vi "vector space kNN.vi"() -> ()   [LabVIEW 2014]
panel:
  out "Numeric":i32
  out "size(s) 2":i32
  out "Results":string[][](array[string])
  out "accuracy":string[][](array[string])
  out "size(s)":i32
  out "Array":string[][](array[string])
  out "appended array":string[](array[string])
  in  "kNN k":i32=5
  out "subarray":dbl[](array[numeric])
  in  "all rows":string[][](array[string])=array2038x3[6114 elements]
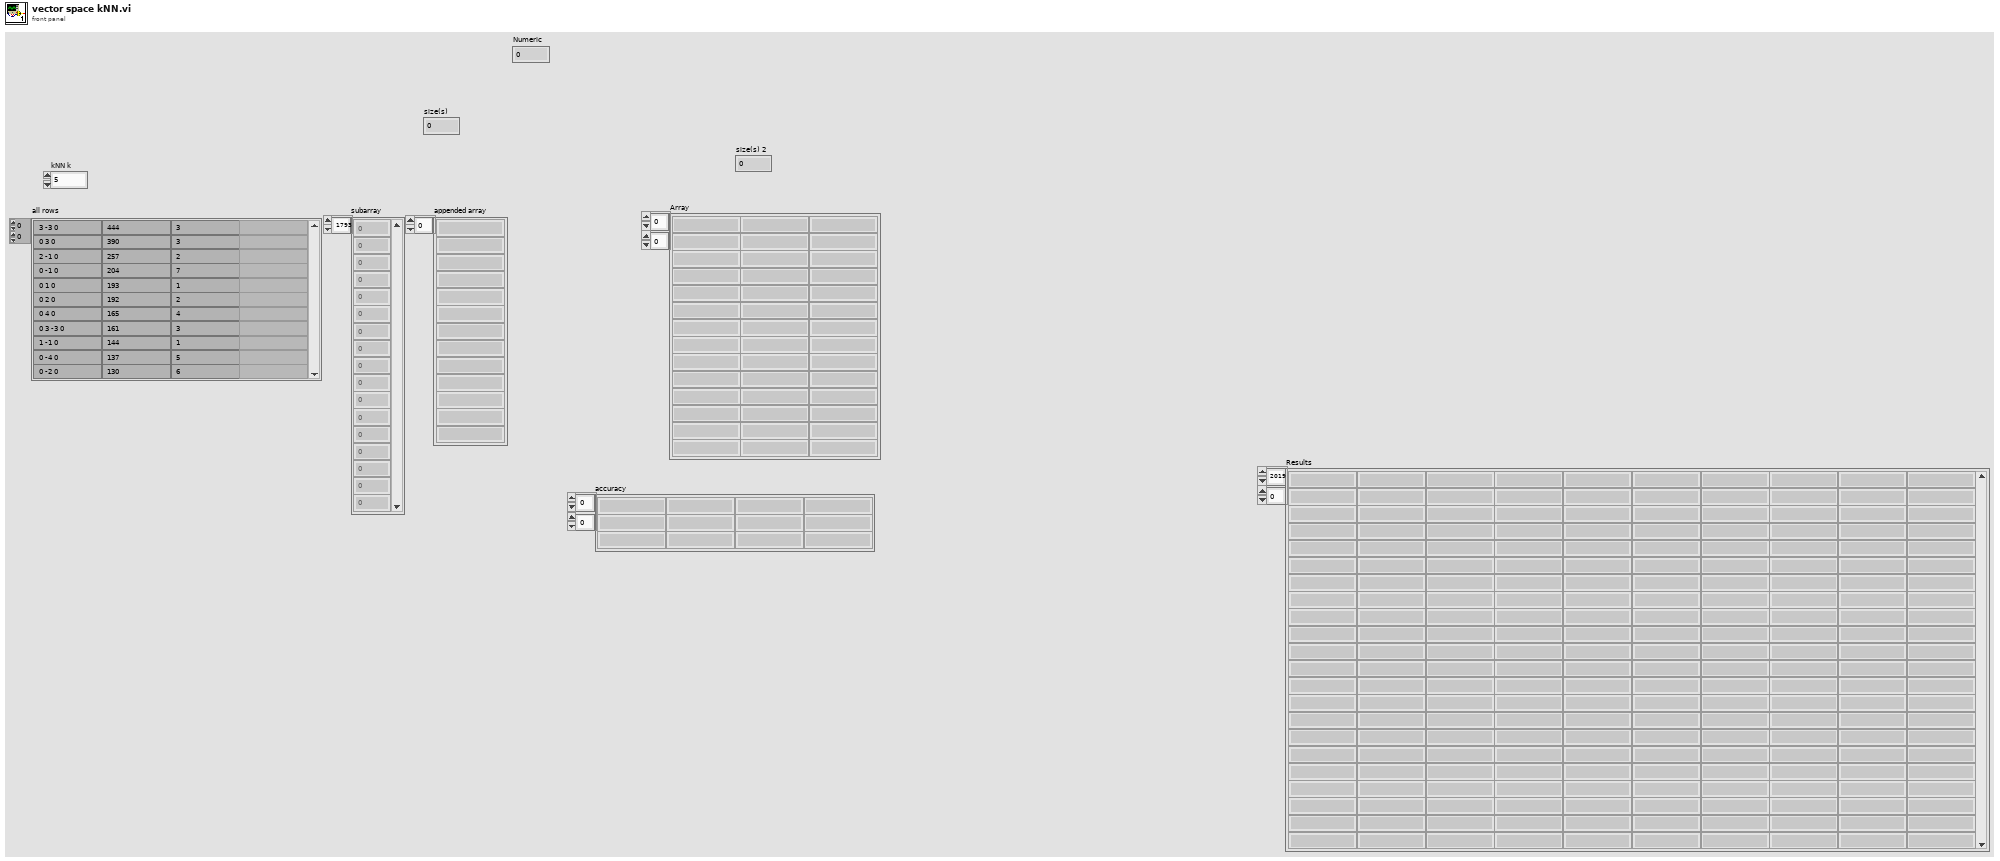
[diagram p1: front panel]
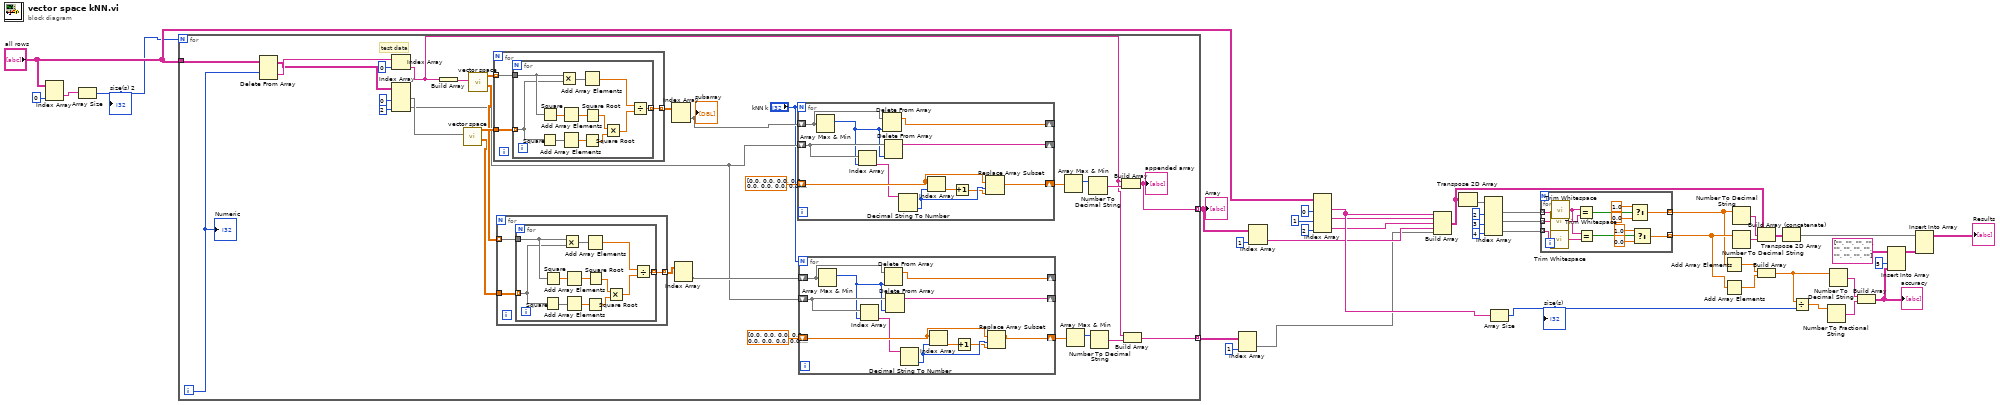
[diagram p0: block diagram]
diagram:
  n1 = Index Array(array="all rows", index (col)=0 ("disabled index (col)")) -> (element=w2:string[])  [unwired: 1 in]
  n2 = Array Size(array=w2) -> (size(s)=w1:i32)
  "size(s) 2" <- w1
  n3 = for {
    N: w1 -> [_]
    tunnel: "all rows" -> [w72]
    tunnel: [w55] -> w9 mode=indexing
    tunnel: [w44] -> w6 mode=indexing
    i -> [w71]
    # "test data"
    n4 = Delete From Array(array=w72, index (row)=w71) -> (deleted portion=w70:string[], array with subset deleted=w67:string[][])  [unwired: 2 in]
    n5 = Index Array(array=w70, index=0 ("disabled index (col)")) -> (element=w45:string)
    n6 = Index Array(array=w67, index (col) #1=0 ("disabled index (col)"), index (col) #2=2 ("index (col)")) -> (element #1=w61:string[], element #2=w46:string[])  [unwired: 2 in]
    n7 = Build Array(w45) -> (w64:string[])
    n8 = call "vector space.vi"("Full transition sequence from service to end"=w61) -> ("vector (directional transitions)"=w52:dbl[][], "vector positions only"=w63:dbl[][])  [unwired: 8 in, 1 out]
    n9 = call "vector space.vi"("Full transition sequence from service to end"=w64) -> ("vector (directional transitions)"=w53:dbl[][], "vector positions only"=w62:dbl[][])  [unwired: 8 in, 1 out]
    n10 = for {
      tunnel: w62 -> [w111] mode=indexing
      tunnel: w63 -> [w112]
      tunnel: [w110] -> w65 mode=indexing
      n11 = for {
        tunnel: w112 -> [w118] mode=indexing
        tunnel: w111 -> [w124]
        tunnel: [w113] -> w110 mode=indexing
        n12 = Square(x=w118) -> (x^2=w119:dbl[])
        n13 = Square(x=w124) -> (x^2=w122:dbl[])
        n14 = Multiply(x=w124, y=w118) -> (x*y=w123:dbl[])
        n15 = Add Array Elements(numeric array=w119) -> (sum=w120:dbl)
        n16 = Add Array Elements(numeric array=w122) -> (sum=w121:dbl)
        n17 = Add Array Elements(numeric array=w123) -> (sum=w114:dbl)
        n18 = Square Root(x=w120) -> (sqrt(x)=w116:dbl)
        n19 = Square Root(x=w121) -> (sqrt(x)=w117:dbl)
        n20 = Multiply(x=w117, y=w116) -> (x*y=w115:dbl)
        n21 = Divide(x=w114, y=w115) -> (x/y=w113:dbl)
      }
    }
    n22 = for {
      tunnel: w53 -> [w85] mode=indexing
      tunnel: w52 -> [w86]
      tunnel: [w84] -> w54 mode=indexing
      n23 = for {
        tunnel: w86 -> [w92] mode=indexing
        tunnel: w85 -> [w98]
        tunnel: [w87] -> w84 mode=indexing
        n24 = Square(x=w92) -> (x^2=w93:dbl[])
        n25 = Square(x=w98) -> (x^2=w96:dbl[])
        n26 = Multiply(x=w98, y=w92) -> (x*y=w97:dbl[])
        n27 = Add Array Elements(numeric array=w93) -> (sum=w94:dbl)
        n28 = Add Array Elements(numeric array=w96) -> (sum=w95:dbl)
        n29 = Add Array Elements(numeric array=w97) -> (sum=w88:dbl)
        n30 = Square Root(x=w94) -> (sqrt(x)=w90:dbl)
        n31 = Square Root(x=w95) -> (sqrt(x)=w91:dbl)
        n32 = Multiply(x=w91, y=w90) -> (x*y=w89:dbl)
        n33 = Divide(x=w88, y=w89) -> (x/y=w87:dbl)
      }
    }
    n34 = Index Array(array=w65) -> (element=w56:dbl[])  [unwired: 2 in]
    "subarray" <- w56
    n35 = Index Array(array=w54) -> (element=w47:dbl[])  [unwired: 2 in]
    n36 = for {
      N: "kNN k" -> [_]
      shift-right: [w106] -> _
      shift-left: w56 -> [w109]
      shift-right: [w105] -> _
      shift-left: w46 -> [w108]
      shift-right: [w100] -> w59
      shift-left: dbl[] [0.0, 0.0, 0.0, 0.0, 0.0, 0.0, 0.0, 0.0, 0.0, 0.0, 0.0, 0.0] -> [w101]
      n37 = Array Max & Min(array=w109) -> (max index (indices)=w107:i32)  [unwired: 3 out]
      n38 = Index Array(array=w108, index=w107) -> (element=w99:string)
      n39 = Delete From Array(array=w109, index=w107) -> (array with subset deleted=w106:dbl[])  [unwired: 1 in, 1 out]
      n40 = Delete From Array(array=w108, index=w107) -> (array with subset deleted=w105:string[])  [unwired: 1 in, 1 out]
      n41 = Decimal String To Number(string=w99) -> (number=w104:i32)  [unwired: 2 in, 1 out]
      n42 = Index Array(array=w101, index=w104) -> (element=w102:dbl)
      n43 = Increment(x=w102) -> (x+1=w103:dbl)
      n44 = Replace Array Subset(array=w101, new element=w103, index=w104) -> (w100:dbl[])
    }
    n45 = for {
      N: "kNN k" -> [_]
      shift-right: [w80] -> _
      shift-left: w47 -> [w83]
      shift-right: [w79] -> _
      shift-left: w46 -> [w82]
      shift-right: [w74] -> w49
      shift-left: dbl[] [0.0, 0.0, 0.0, 0.0, 0.0, 0.0, 0.0, 0.0, 0.0, 0.0, 0.0, 0.0] -> [w75]
      n46 = Array Max & Min(array=w83) -> (max index (indices)=w81:i32)  [unwired: 3 out]
      n47 = Index Array(array=w82, index=w81) -> (element=w73:string)
      n48 = Delete From Array(array=w83, index=w81) -> (array with subset deleted=w80:dbl[])  [unwired: 1 in, 1 out]
      n49 = Delete From Array(array=w82, index=w81) -> (array with subset deleted=w79:string[])  [unwired: 1 in, 1 out]
      n50 = Decimal String To Number(string=w73) -> (number=w78:i32)  [unwired: 2 in, 1 out]
      n51 = Index Array(array=w75, index=w78) -> (element=w76:dbl)
      n52 = Increment(x=w76) -> (x+1=w77:dbl)
      n53 = Replace Array Subset(array=w75, new element=w77, index=w78) -> (w74:dbl[])
    }
    n54 = Array Max & Min(array=w59) -> (max index (indices)=w58:i32)  [unwired: 3 out]
    n55 = Array Max & Min(array=w49) -> (max index (indices)=w50:i32)  [unwired: 3 out]
    n56 = Number To Decimal String(number=w58) -> (decimal integer string=w60:string)  [unwired: 1 in]
    n57 = Number To Decimal String(number=w50) -> (decimal integer string=w48:string)  [unwired: 1 in]
    n58 = Build Array(w45, w60) -> (w55:string[])
    "appended array" <- w55
    n59 = Build Array(w45, w48) -> (w44:string[])
    "Numeric" <- w71
  }
  "Array" <- w9
  n60 = Index Array(array=w6, index (col)=1 ("disabled index (col)")) -> (element=w5:string[])  [unwired: 1 in]
  n61 = Index Array(array=w9, index (col)=1 ("disabled index (col)")) -> (element=w8:string[])  [unwired: 1 in]
  n62 = Index Array(array="all rows", index (col) #1=0 ("disabled index (col)"), index (col) #2=1 ("index (col)"), index (col) #3=2 ("index (col)")) -> (element #1=w41:string[], element #2=w37:string[], element #3=w38:string[])  [unwired: 3 in]
  n63 = Build Array(w41, w37, w38, w8, w5) -> (w40:string[][])
  n64 = Transpose 2D Array(2D array=w40) -> (transposed array=w19:string[][])
  n65 = Index Array(array=w19, index (col) #1=2 ("disabled index (col)"), index (col) #2=3 ("index (col)"), index (col) #3=4 ("index (col)")) -> (element #1=w16:string[], element #2=w17:string[], element #3=w18:string[])  [unwired: 3 in]
  n66 = Array Size(array=w41) -> (size(s)=w42:i32)
  "size(s)" <- w42
  n67 = for {
    tunnel: w16 -> [w130] mode=indexing
    tunnel: w17 -> [w129] mode=indexing
    tunnel: w18 -> [w128] mode=indexing
    tunnel: [w132] -> w34 mode=indexing
    tunnel: [w131] -> w35 mode=indexing
    n68 = call <vilib>:"Trim Whitespace.vi"("string"=w129) -> ("trimmed string"=w127:string)  [unwired: 1 in]
    n69 = call <vilib>:"Trim Whitespace.vi"("string"=w128) -> ("trimmed string"=w126:string)  [unwired: 1 in]
    n70 = call <vilib>:"Trim Whitespace.vi"("string"=w130) -> ("trimmed string"=w125:string)  [unwired: 1 in]
    n71 = Equal?(x=w125, y=w127) -> (x = y?=w138:bool)
    n72 = Equal?(x=w125, y=w126) -> (x = y?=w133:bool)
    n73 = Select(t=1.0, s=w138, f=0.0) -> (s? t:f=w132:dbl)
    n74 = Select(t=1.0, s=w133, f=0.0) -> (s? t:f=w131:dbl)
  }
  n75 = Add Array Elements(numeric array=w34) -> (sum=w33:dbl)
  n76 = Add Array Elements(numeric array=w35) -> (sum=w32:dbl)
  n77 = Number To Decimal String(number=w34) -> (decimal integer string=w20:string[])  [unwired: 1 in]
  n78 = Number To Decimal String(number=w35) -> (decimal integer string=w21:string[])  [unwired: 1 in]
  n79 = Build Array (concatenate)(w40, w20, w21) -> (w22:string[][])
  n80 = Build Array(w33, w32) -> (w31:dbl[])
  n81 = Transpose 2D Array(2D array=w22) -> (transposed array=w36:string[][])
  n82 = Divide(x=w31, y=w42) -> (x/y=w30:dbl[])
  n83 = Number To Fractional String(number=w30) -> (F-format string=w28:string[])  [unwired: 3 in]
  n84 = Number To Decimal String(number=w31) -> (decimal integer string=w29:string[])  [unwired: 1 in]
  n85 = Build Array(w29, w28) -> (w24:string[][])
  "accuracy" <- w24
  n86 = Insert Into Array(array=string[][] [["", "", "", "", "", ""], ["", "", "", "", "", ""]] ("appended array 3"), index (col)=5 ("disabled index (col)"), new element=w24) -> (w25:string[][])  [unwired: 1 in]
  n87 = Insert Into Array(array=w36, new element=w25) -> (→"Results":string[][])  [unwired: 2 in]
